vi "CRYGet Wave File Information.vi"(0 "FileNameStr":string="I:\\__From JASON\\20141011_sound\\pink_noise_44100_filtered.wav") -> (4 "sound format":T1={"sample rate (S/s)"=22050.0, "number of channels"=2, "bits per sample"=16}, 6 "wave info":T2={"total number of samples/ch"=16, "total byte number"=2, "Time DBL"=0.0, "format str"="", "Time Str"="", "peak FSD"=0.0, "rms FSD"=0.0, "peak %FSD"=0.0, "rms %FSD"=0.0, "rms"=0.0, "Channel Number"=0, "rms L"=0.0, "rms R"=0.0}, 8 "wave data out":i32[](array[numeric]), 15 "Error Output":errorcluster)   [LabVIEW 2013]
uses:
  Typedef Control/CRYWaveFile Information Typedef.ctl
  <vilib>/sound2/lvsound2.llb/Sound Data Format.ctl
  <vilib>/Analysis/5stat.llb/RMS (DBL).vi
  <vilib>/Analysis/NI_AALPro.lvlib
  CRYSound.dll
panel:
  out "Waveform Graph 2":dbl[](graph)
  out "waveformattag":i32
  out "Waveform Graph":dbl[](graph)
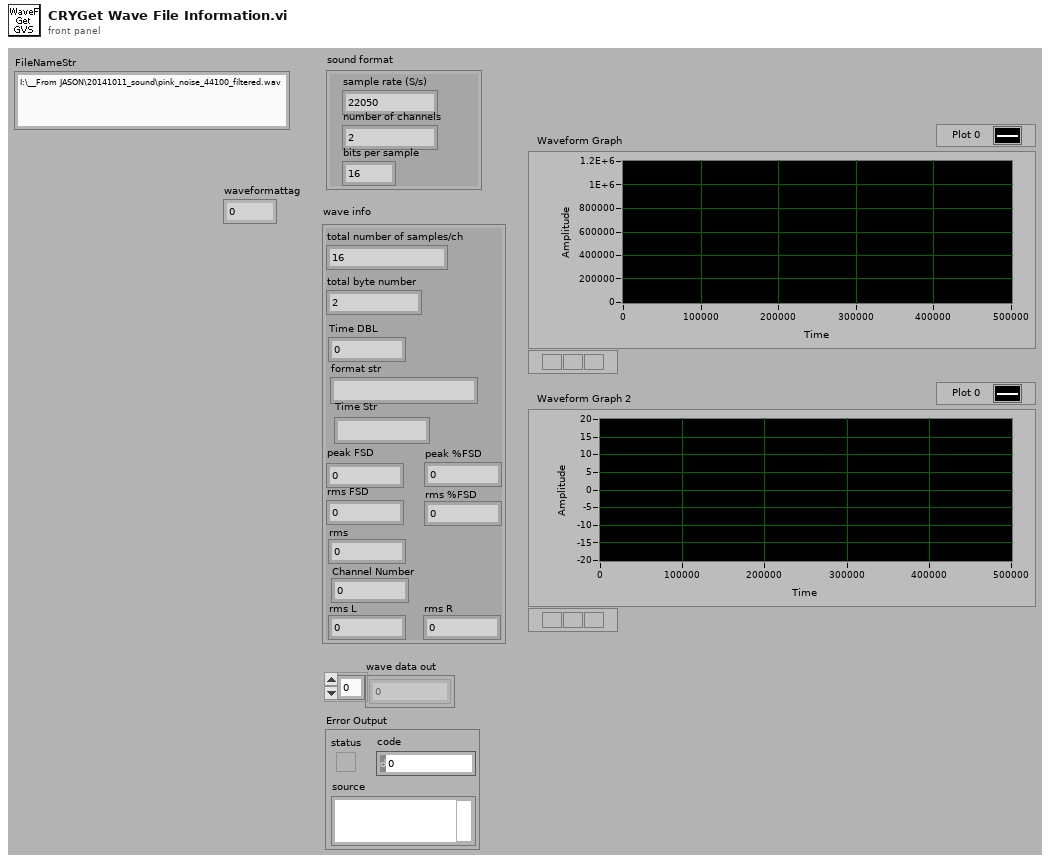
[diagram p1: front panel]
types:
  T1 = typedef "Sound Data Format.ctl" = cluster{"sample rate (S/s)":dbl, "number of channels":i32, "bits per sample":i32}
  T2 = typedef "CRYWaveFile Information Typedef.ctl" = cluster{"total number of samples/ch":u32, "total byte number":u32, "Time DBL":dbl, "format str":string, "Time Str":string, "peak FSD":dbl, "rms FSD":dbl, "peak %FSD":dbl, "rms %FSD":dbl, "rms":dbl, "Channel Number":u16, "rms L":dbl, "rms R":dbl}
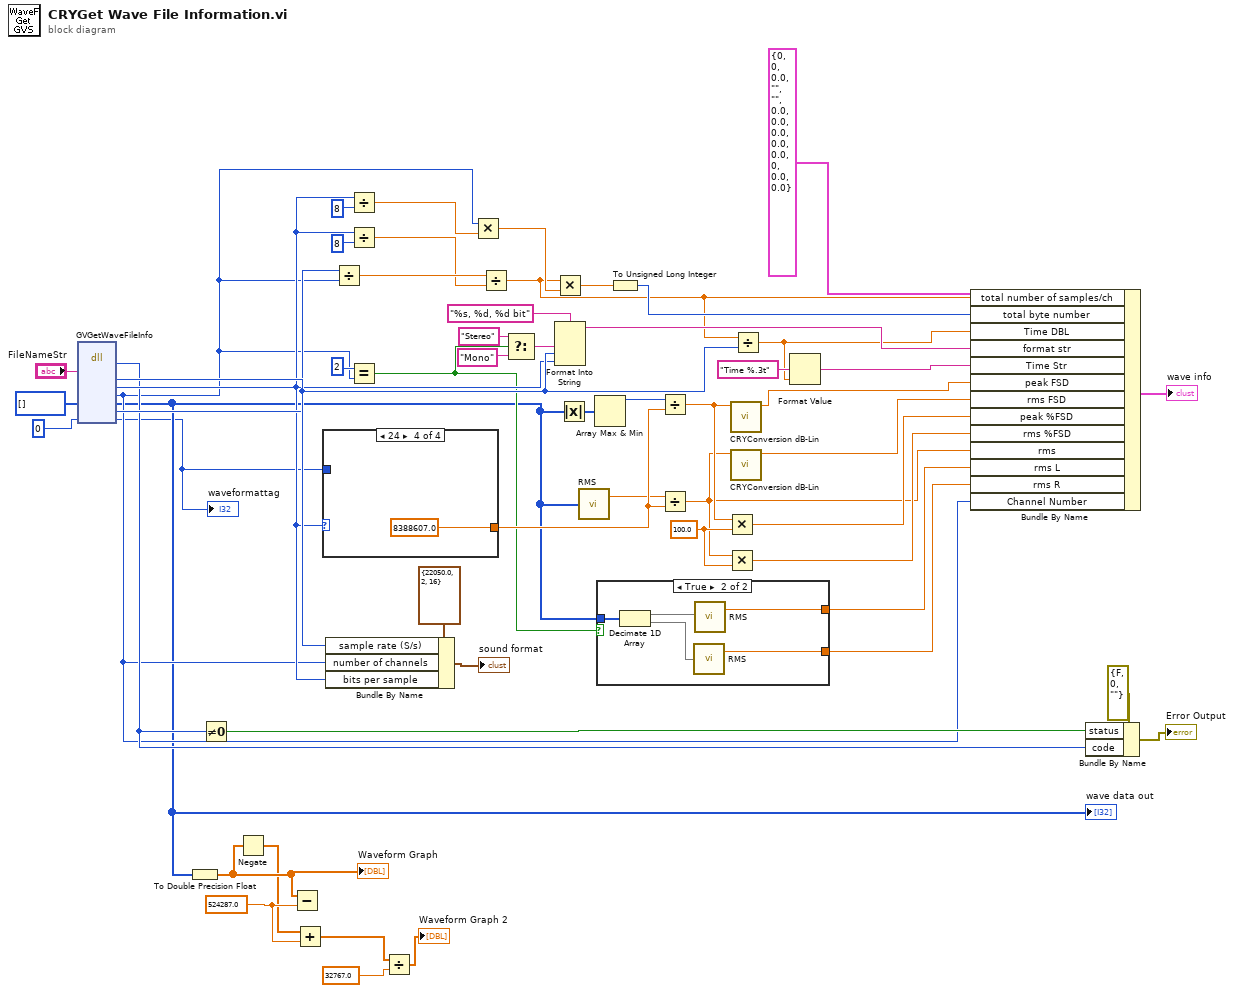
[diagram p0: block diagram]
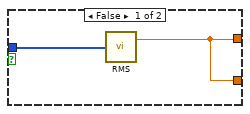
[diagram p2: hidden frame]
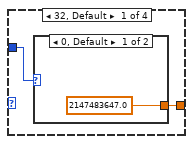
[diagram p3: hidden frame]
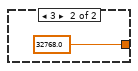
[diagram p4: hidden frame]
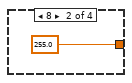
[diagram p5: hidden frame]
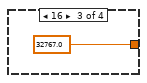
[diagram p6: hidden frame]
diagram:
  w5 = 524287.0 ("y")
  w28 = 100.0 ("y")
  n1 = dll-call lib="D:/LabView_Project/CRY6181/CRYSound.dll" fn="GVGetWaveFileInfo"("FileName"="FileNameStr", "pSampleData"=i32[] [] ("noise"), "waveformattag"=0) -> ("return type"=w47:u32, "SampleFreq"=w54:u32, "BitDepth"=w52:u32, "nChannels"=w10:u32, "pSampleData"=w9:i32[], "nDataLen"=w53:i32, "waveformattag"=w7:i32)  [unwired: 4 in, 6 out]
  "wave data out" <- w9
  "waveformattag" <- w7
  n2 = To Double Precision Float(number=w9) -> (double precision float=w6:dbl[])
  "Waveform Graph" <- w6
  n3 = Not Equal To 0?(x=w47) -> (x != 0?=w48:bool)
  n4 = Negate(x=w6) -> (-x=w4:dbl[])
  n5 = Subtract(x=w6, y=w5) -> ()  [unwired: 1 out]
  n6 = Add(x=w4, y=w5) -> (x+y=w2:dbl[])
  n7 = case shown="24" w52 {
    tunnel: [w57 255.0 ("y") 32767.0 ("y") 8388607.0 ("y")] -> w15
    tunnel: w7 -> [w56 _ _ _]
    frame 32, Default {
      n8 = case shown="0, Default" w56 {
        tunnel: [2147483647.0 ("y") 32768.0 ("y")] -> w57
        frame 0, Default {
        }
        frame 3 {
        }
      }
    }
    frame 8 {
    }
    frame 16 {
    }
    frame 24 {
    }
  }
  n9 = Bundle By Name(cluster=T1 {"sample rate (S/s)"=22050.0, "number of channels"=2, "bits per sample"=16} ("sound format"), "sample rate (S/s)"=w54, "number of channels"=w10, "bits per sample"=w52) -> (→"sound format":T1)
  n10 = Divide(x=w53, y=w10) -> (x/y=w25:dbl)
  n11 = Divide(x=w52, y=u32 8) -> (x/y=w44:dbl)
  n12 = Divide(x=w52, y=i16 8) -> (x/y=w23:dbl)
  n13 = Equal?(x=2 ("y"), y=w10) -> (x = y?=w13:bool)
  n14 = Divide(x=w2, y=32767.0) -> (x/y=→"Waveform Graph 2":dbl[])
  n15 = Multiply(x=w10, y=w44) -> (x*y=w46:dbl)
  n16 = Divide(x=w25, y=w23) -> (x/y=w22:dbl)
  n17 = Select(t="Stereo" ("format string"), s=w13, f="Mono" ("format string")) -> (s? t:f=w42:string)
  n18 = Multiply(x=w22, y=w46) -> (x*y=w38:dbl)
  n19 = Format Into String(format string="%s, %d, %d bit", w42, w54, w52) -> (resulting string=w35:string)  [unwired: 2 in, 1 out]
  n20 = Absolute Value(x=w9) -> (abs(x)=w20:i32[])
  n21 = call-poly <vilib>:"RMS.vi"("X"=w9) -> ("rms value"=w14:dbl)  [unwired: 1 out]
  n22 = Array Max & Min(array=w20) -> (max value=w21:i32)  [unwired: 3 out]
  n23 = case shown="True" w13 {
    tunnel: w9 -> [w64 w69]
    tunnel: [w63 w66] -> w12
    tunnel: [w63 w65] -> w11
    frame False {
      n24 = call-poly <vilib>:"RMS.vi"("X"=w64) -> ("rms value"=w63:dbl)  [unwired: 1 out]
    }
    frame True {
      n25 = Decimate 1D Array(w69) -> (w68:i32[], w67:i32[])
      n26 = call-poly <vilib>:"RMS.vi"("X"=w67) -> ("rms value"=w65:dbl)  [unwired: 1 out]
      n27 = call-poly <vilib>:"RMS.vi"("X"=w68) -> ("rms value"=w66:dbl)  [unwired: 1 out]
    }
  }
  n28 = To Unsigned Long Integer(number=w38) -> (unsigned 32bit integer=w37:u32)
  n29 = Divide(x=w21, y=w15) -> (x/y=w18:dbl)
  n30 = Divide(x=w14, y=w15) -> (x/y=w16:dbl)
  n31 = Multiply(x=w18, y=w28) -> (x*y=w30:dbl)
  n32 = Multiply(x=w16, y=w28) -> (x*y=w29:dbl)
  n33 = call "CRYConversion dB-Lin.vi"("Lin In"=w18) -> ("Log Out"=w17:dbl)  [unwired: 5 in, 3 out]
  n34 = call "CRYConversion dB-Lin.vi"("Lin In"=w16) -> ("Log Out"=w19:dbl)  [unwired: 5 in, 3 out]
  n35 = Divide(x=w22, y=w54) -> (x/y=w33:dbl)
  n36 = Format Value(format string="Time %.3t" ("time format string (%c)"), value (0)=w33) -> (output string=w36:string)  [unwired: 1 out]
  n37 = Bundle By Name(cluster=T2 {"total number of samples/ch"=0, "total byte number"=0, "Time DBL"=0.0, "format str"="", "Time Str"="", "peak FSD"=0.0, "rms FSD"=0.0, "peak %FSD"=0.0, "rms %FSD"=0.0, "rms"=0.0, "Channel Number"=0, "rms L"=0.0, "rms R"=0.0} ("wave info"), "total number of samples/ch"=w22, "total byte number"=w37, "Time DBL"=w33, "format str"=w35, "Time Str"=w36, "peak FSD"=w17, "rms FSD"=w19, "peak %FSD"=w30, "rms %FSD"=w29, "rms"=w16, "rms L"=w12, "rms R"=w11, "Channel Number"=w10) -> (→"wave info":T2)
  n38 = Bundle By Name(cluster=errorcluster {"status"=FALSE, "code"=0, "source"=""} ("error IO"), "status"=w48, "code"=w47) -> (→"Error Output":errorcluster)
